vi "Alligent.vi"() -> ()   [LabVIEW 2018]
uses:
  <vilib>/userdefined/High Color/IMAQdx.ctl
  <vilib>/Utility/miscctls.llb/LVRowAndColumnTypeDef.ctl
  <vilib>/vision/driver/NI_Vision_Acquisition_Software.lvlib
  <vilib>/vision/NI_Vision_Development_Module.lvlib
panel:
  out "Centroid":cluster{"X Centroid":sgl, "Y Centroid":sgl} {"Y Centroid" format="%.2f"; "X Centroid" format="%.2f"}
  in  "观察位置":bool
  in  "记录位置":bool
  out "运行提示":string
  in  "相机曝光时间/ms":dbl(slide) scale=0.0..1000.0
  in  "俯仰":cluster{"前进0.1":bool, "后退0.1":bool, "目标位置":dbl} {"目标位置" max=0.0}
  in  "Z":cluster{"前进1mm":bool, "后退1mm":bool, "目标位置":dbl} {"目标位置" max=0.0}
  in  "Y":cluster{"前进1mm":bool, "后退1mm":bool, "目标位置":dbl} {"目标位置" max=0.0}
  in  "X":cluster{"前进1mm":bool, "后退1mm":bool, "目标位置":dbl} {"目标位置" max=0.0}
  in  "退出":bool
  in  "衰减挡位":T1 scale=0.0..3.0
  out "激光器状态":i32[](listbox)
  in  "初始位置":bool
  in  "链接电机":bool
  in  "链接相机":bool
  out "近场图":T2(plugin-control)
  in  "旋转":T3 {"目标位置" max=0.0}
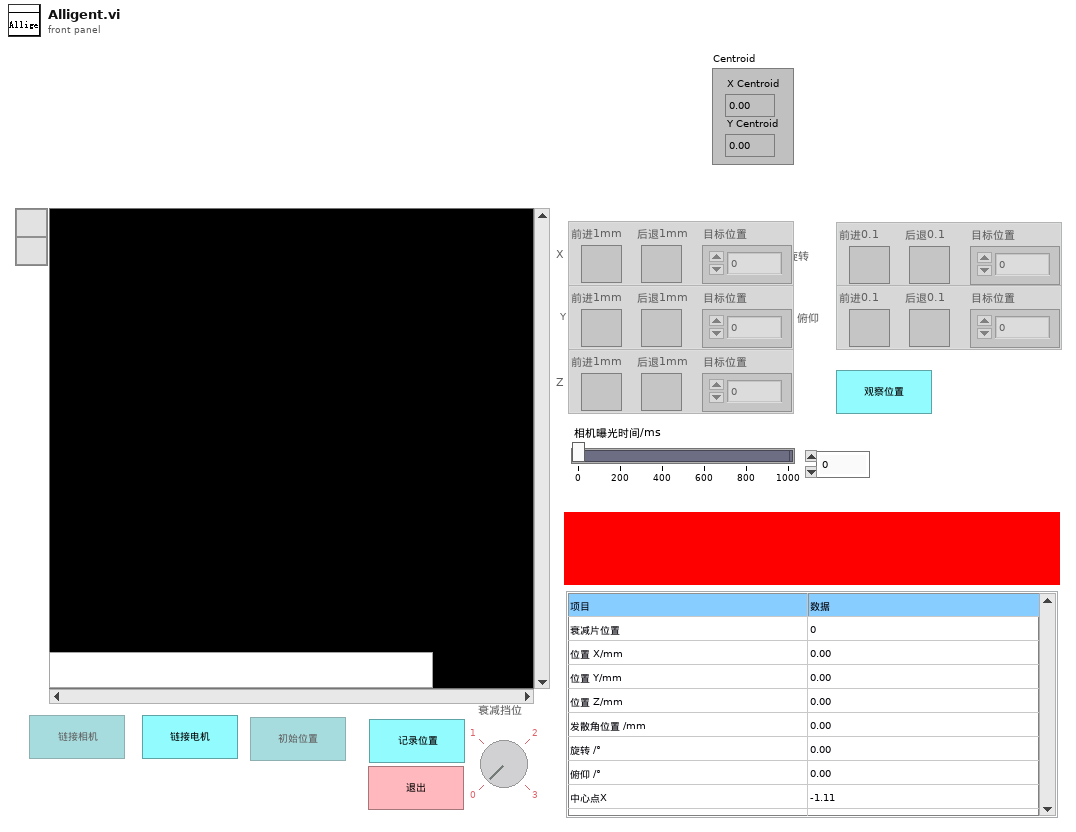
[diagram p1: front panel]
types:
  T1 = typedef "衰减片前面板.ctl" = u8
  T2 = typedef "IMAQ Image.ctl" = refnum<image>
  T3 = typedef "位置调整控件.ctl" = cluster{"前进0.1":bool, "后退0.1":bool, "目标位置":dbl}
  T4 = typedef "IMAQdx.ctl" = refnum<k21>
  T5 = cluster{"链接相机":refnum<vi>, "链接电机":refnum<vi>, "初始位置":refnum<vi>, "退出":refnum<vi>, "衰减挡位":refnum<vi>, "相机曝光时间/ms":refnum<vi>}
  T6 = cluster{"X":refnum<vi>, " Y":refnum<vi>, "Z":refnum<vi>, "  旋转":refnum<vi>, "俯仰":refnum<vi>, "观察位置":refnum<vi>}
  T7 = typedef "衰减片电机位置枚举器.ctl" = enum16{"0倍", "10倍", "100倍", "1000倍"}
  T8 = enum8{"Enabled", "Disabled", "Disabled and Grayed Out"}
  T9 = typedef "衰减片电机指令枚举器.ctl" = enum16{"归0", "停止", "运动", "轴设置", "通信连接", "读取位置"}
  T10 = typedef "控制电机指令枚举器.ctl" = enum16{"归0", "停止", "运动", "轴设置", "通信连接"}
  T11 = typedef "衰减片电机枚举.ctl" = enum16{"小积分球衰减", "偏振仪衰减", "近场相机衰减", "远场相机衰减"}
  T12 = typedef "控制电机位置枚举器.ctl" = enum16{"远场扫描", "发散角扫描", "远场相机", "近场相机", "时间波形", "偏振", "能量", "功率", "光谱"}
  T13 = typedef "控制电机枚举器.ctl" = enum16{"Z", "Y", "X", "发散角", "俯仰", "旋转"}
  T14 = cluster{"激光器型号":string, "X":dbl, "Y":dbl, "Z":dbl, "Rotate":dbl, "Pitching":dbl, "DivergeAngle":dbl, "衰减片位置":cluster{"小积分球位置":T7, "偏振仪位置 ":T7, "近场相机位置 ":T7, "远场相机位置":T7}, "Type":string, "Serial":string}
  T15 = cluster{"远场相机":cluster{"控制电机":T13, "位置":dbl}[], "近场相机":cluster{"控制电机":T13, "位置":dbl}[], "时间波形":cluster{"控制电机":T13, "位置":dbl}[], "偏振":cluster{"控制电机":T13, "位置":dbl}[], "能量":cluster{"控制电机":T13, "位置":dbl}[], "功率":cluster{"控制电机":T13, "位置":dbl}[], "光谱":cluster{"控制电机":T13, "位置":dbl}[], "准直光焦点":cluster{"控制电机":T13, "位置":dbl}[]}
  T16 = typedef "LVRowAndColumnTypeDef.ctl" = cluster{"Row":i32, "Column":i32}
  T17 = cluster{cluster{"控制电机":T13, "NewVal":dbl}, "CMD":string}
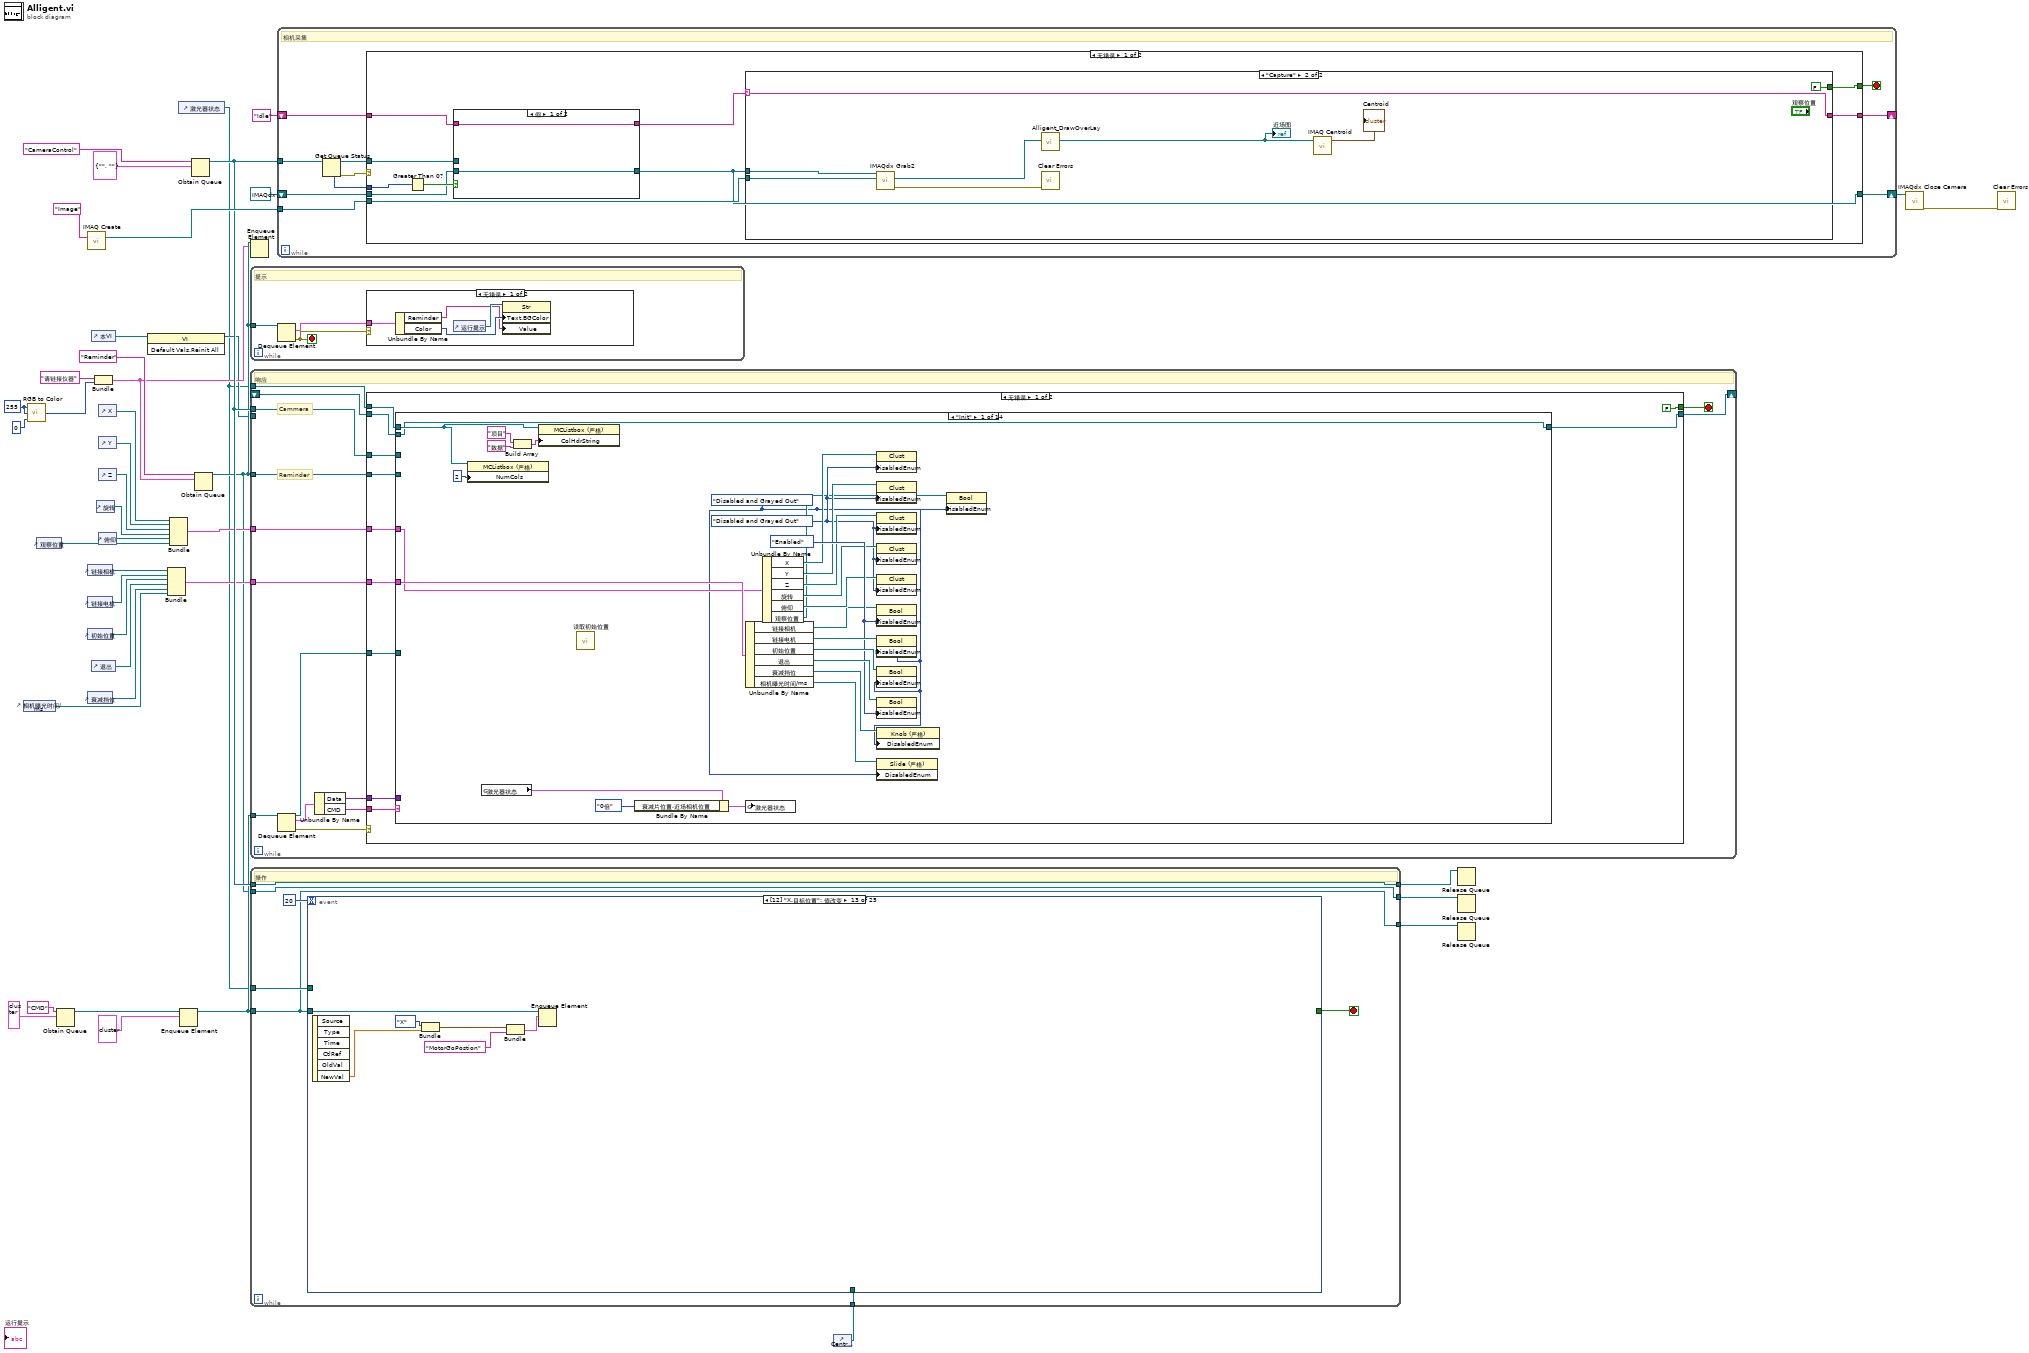
[diagram p0: block diagram]
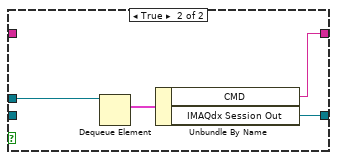
[diagram p3: hidden frame]
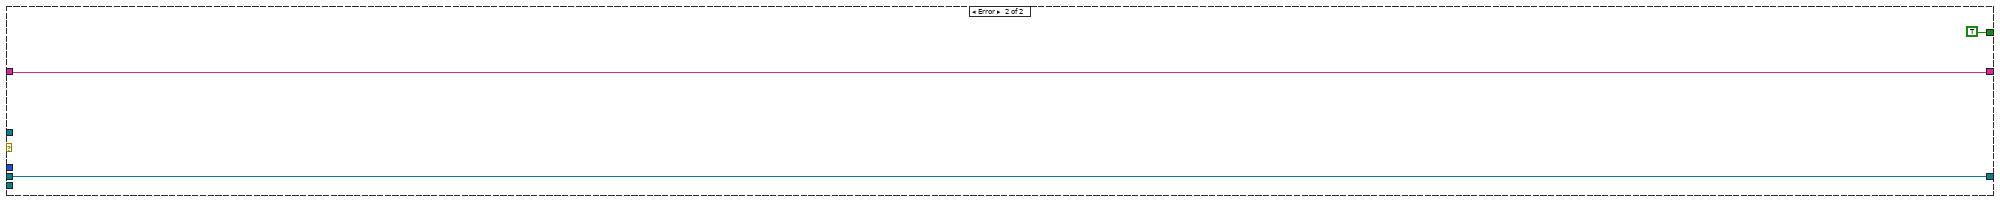
[diagram p5: hidden frame]
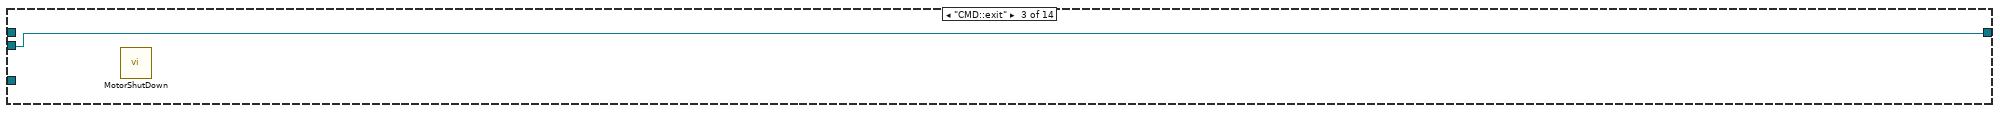
[diagram p7: hidden frame]
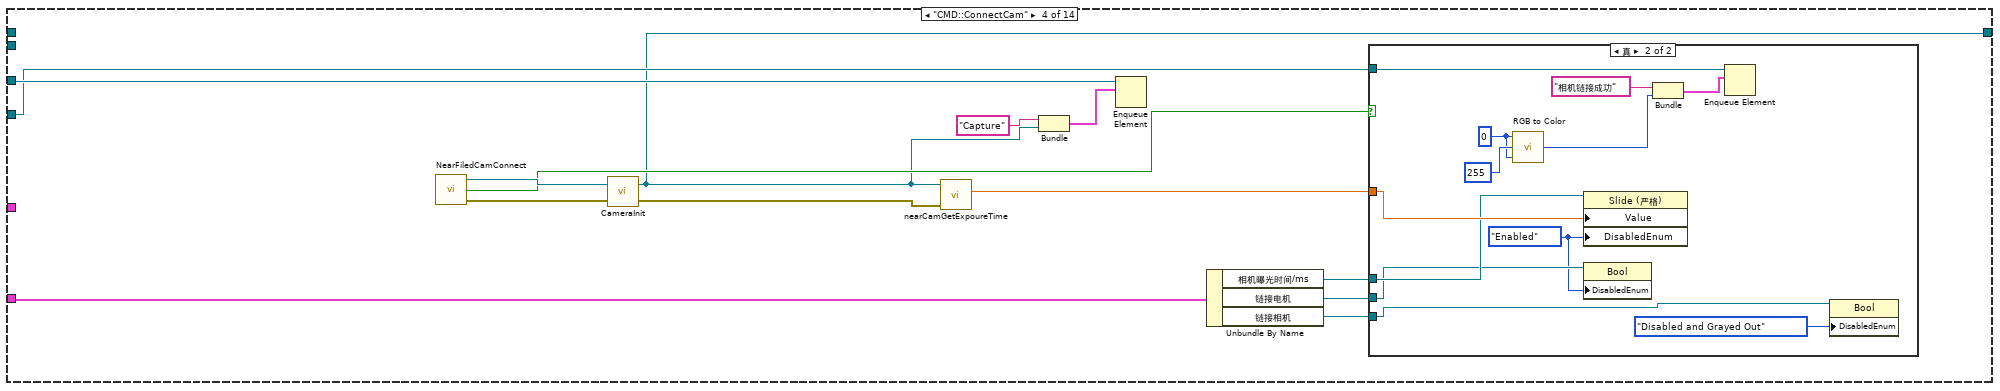
[diagram p8: hidden frame]
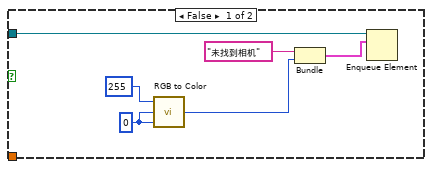
[diagram p9: hidden frame]
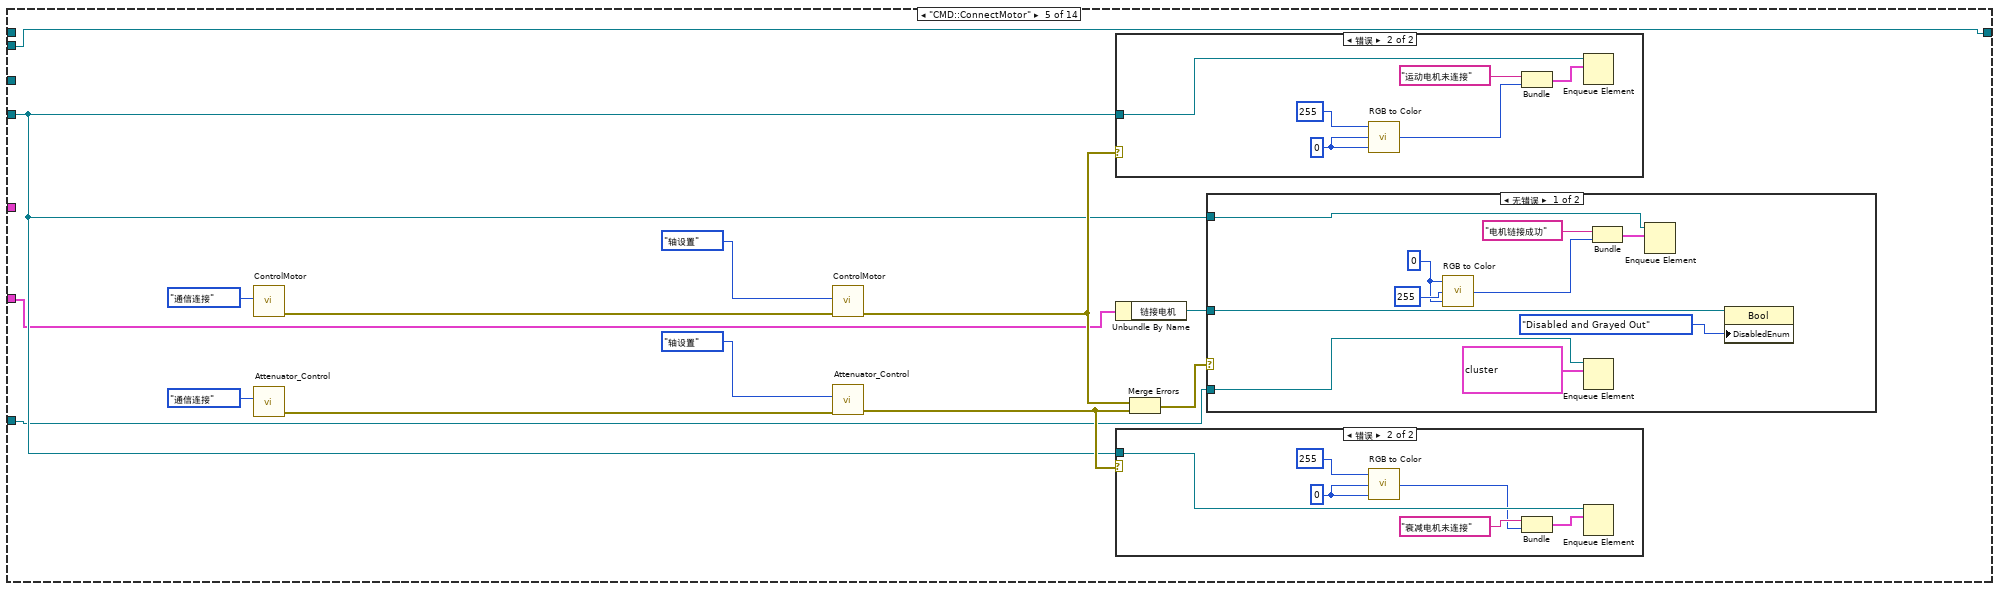
[diagram p10: hidden frame]
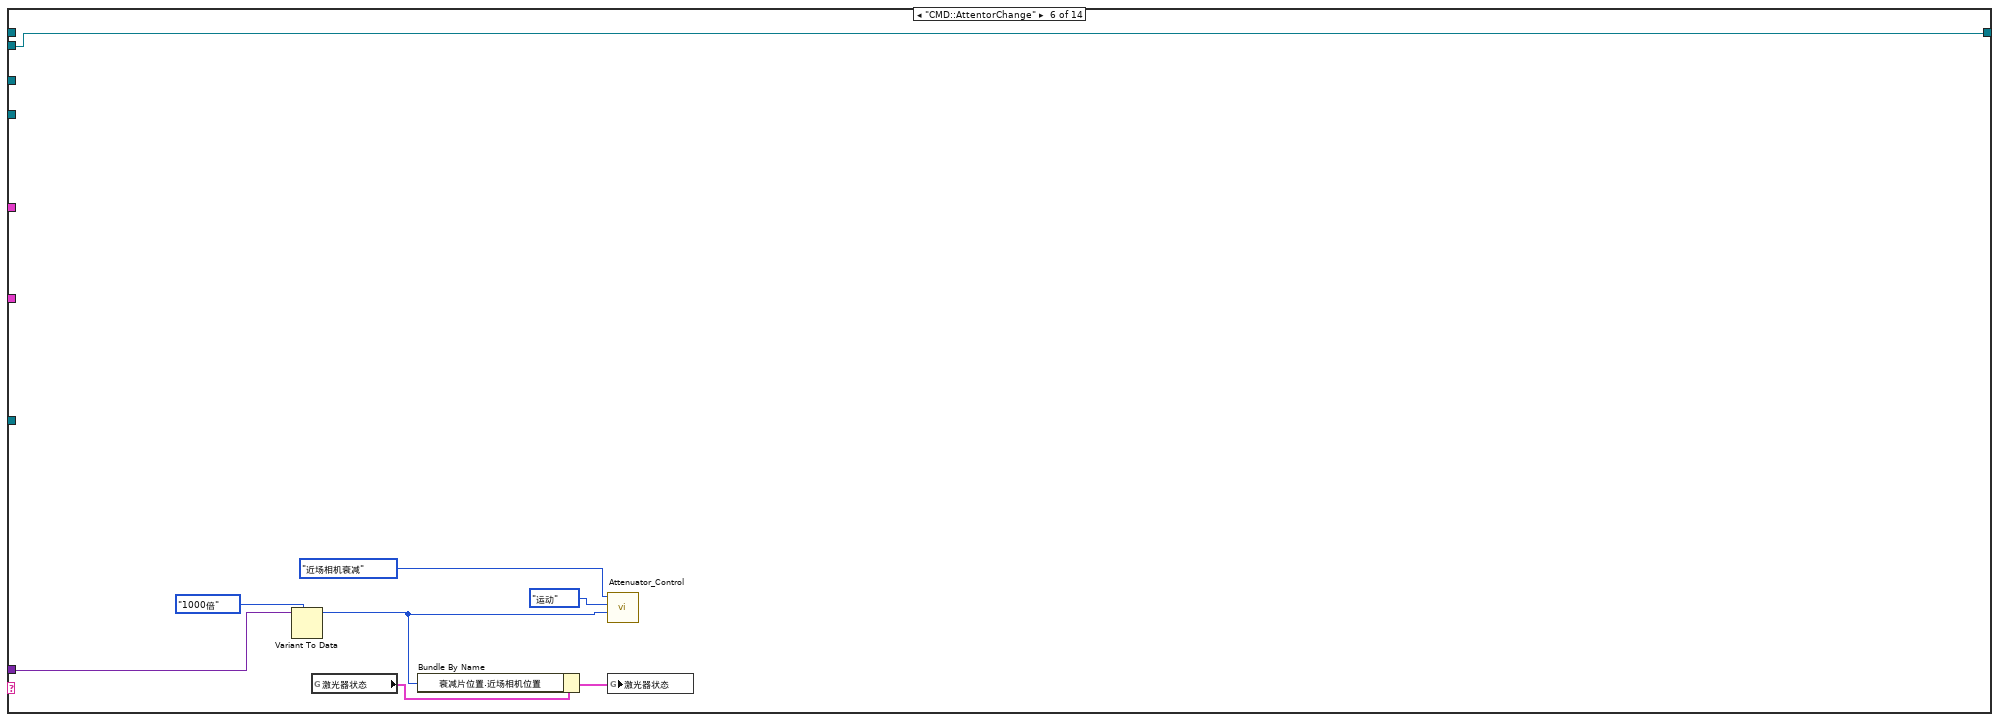
[diagram p14: hidden frame]
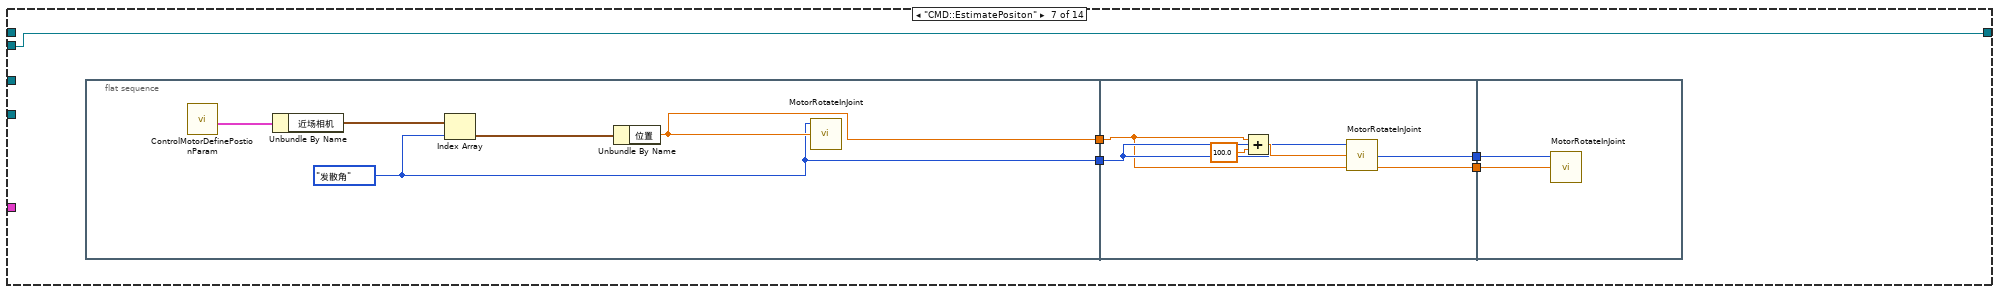
[diagram p15: hidden frame]
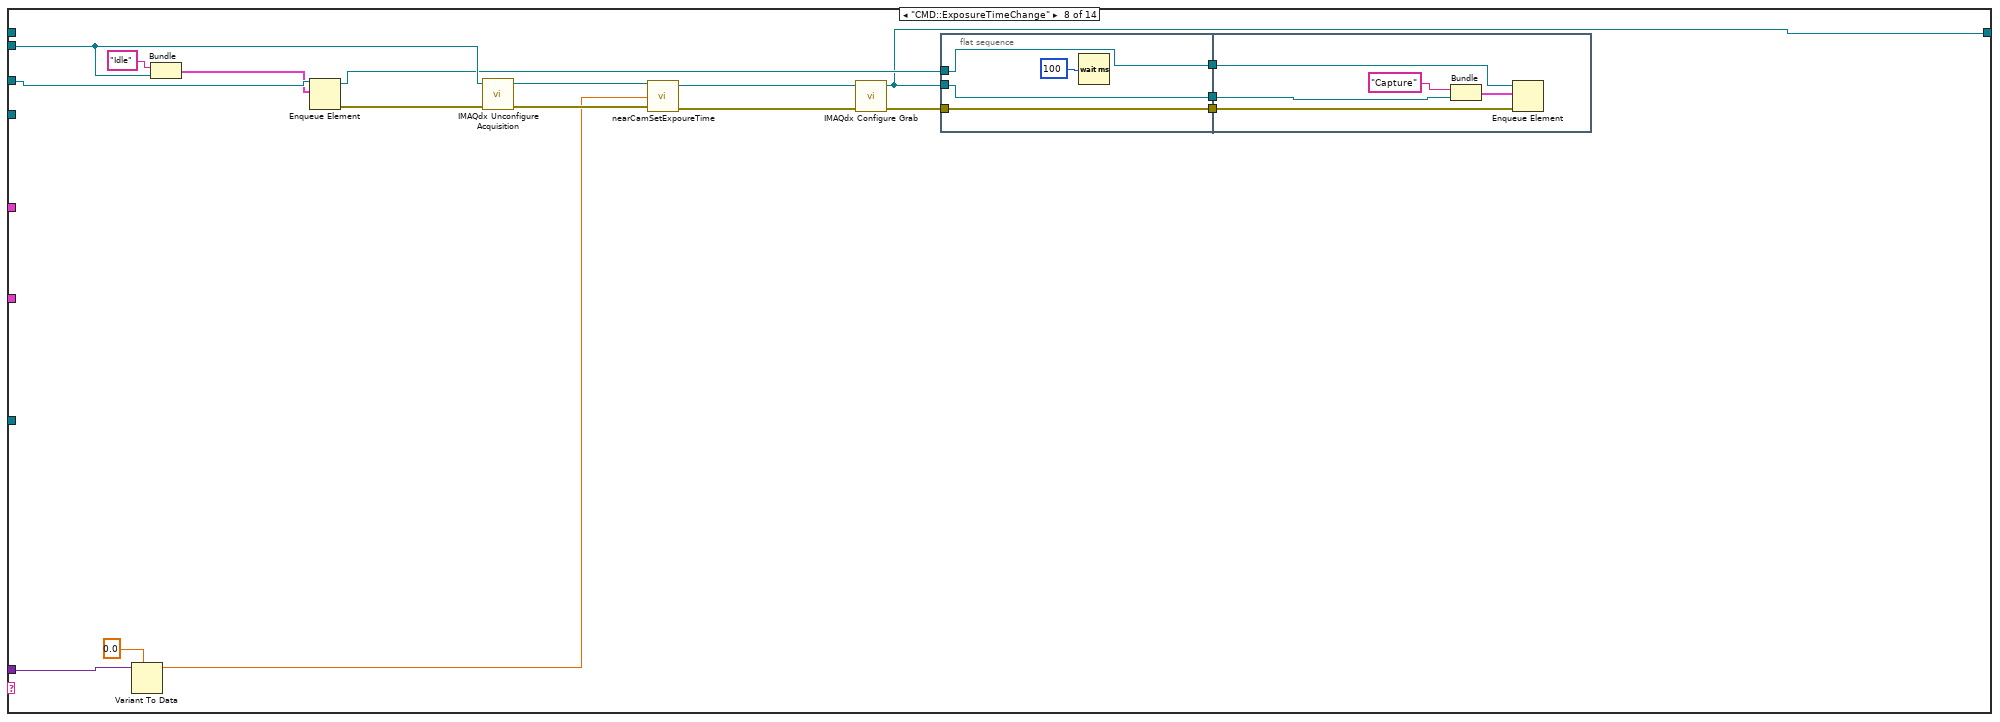
[diagram p16: hidden frame]
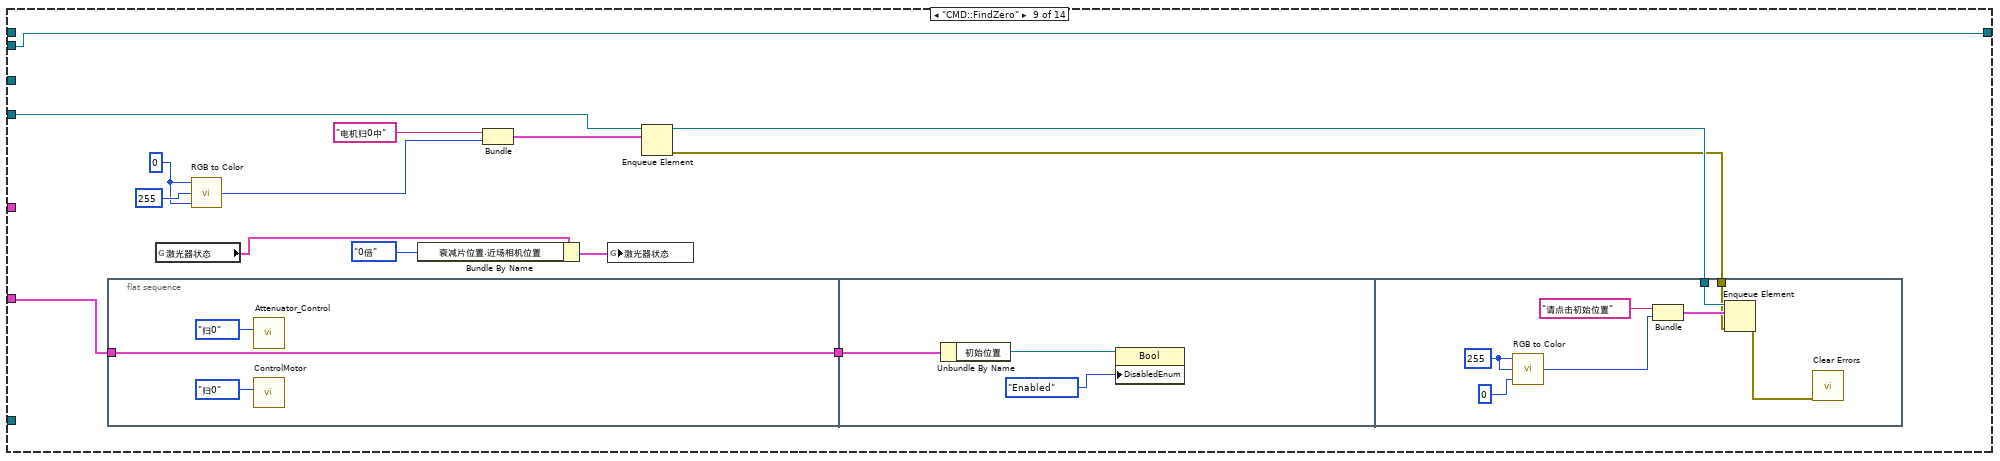
[diagram p17: hidden frame]
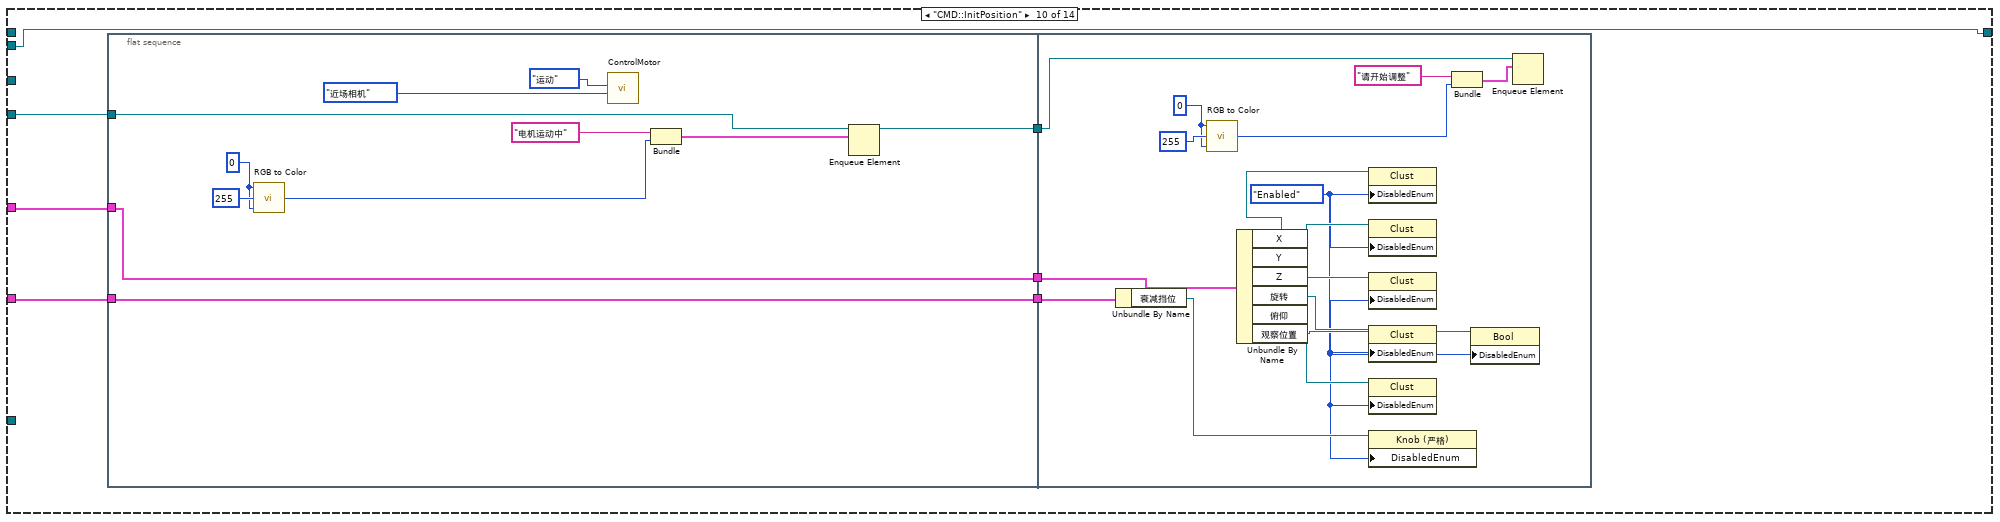
[diagram p18: hidden frame]
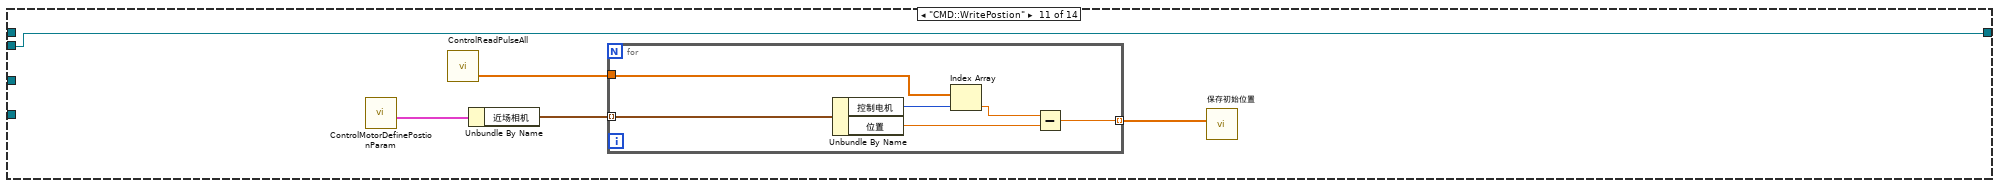
[diagram p19: hidden frame]
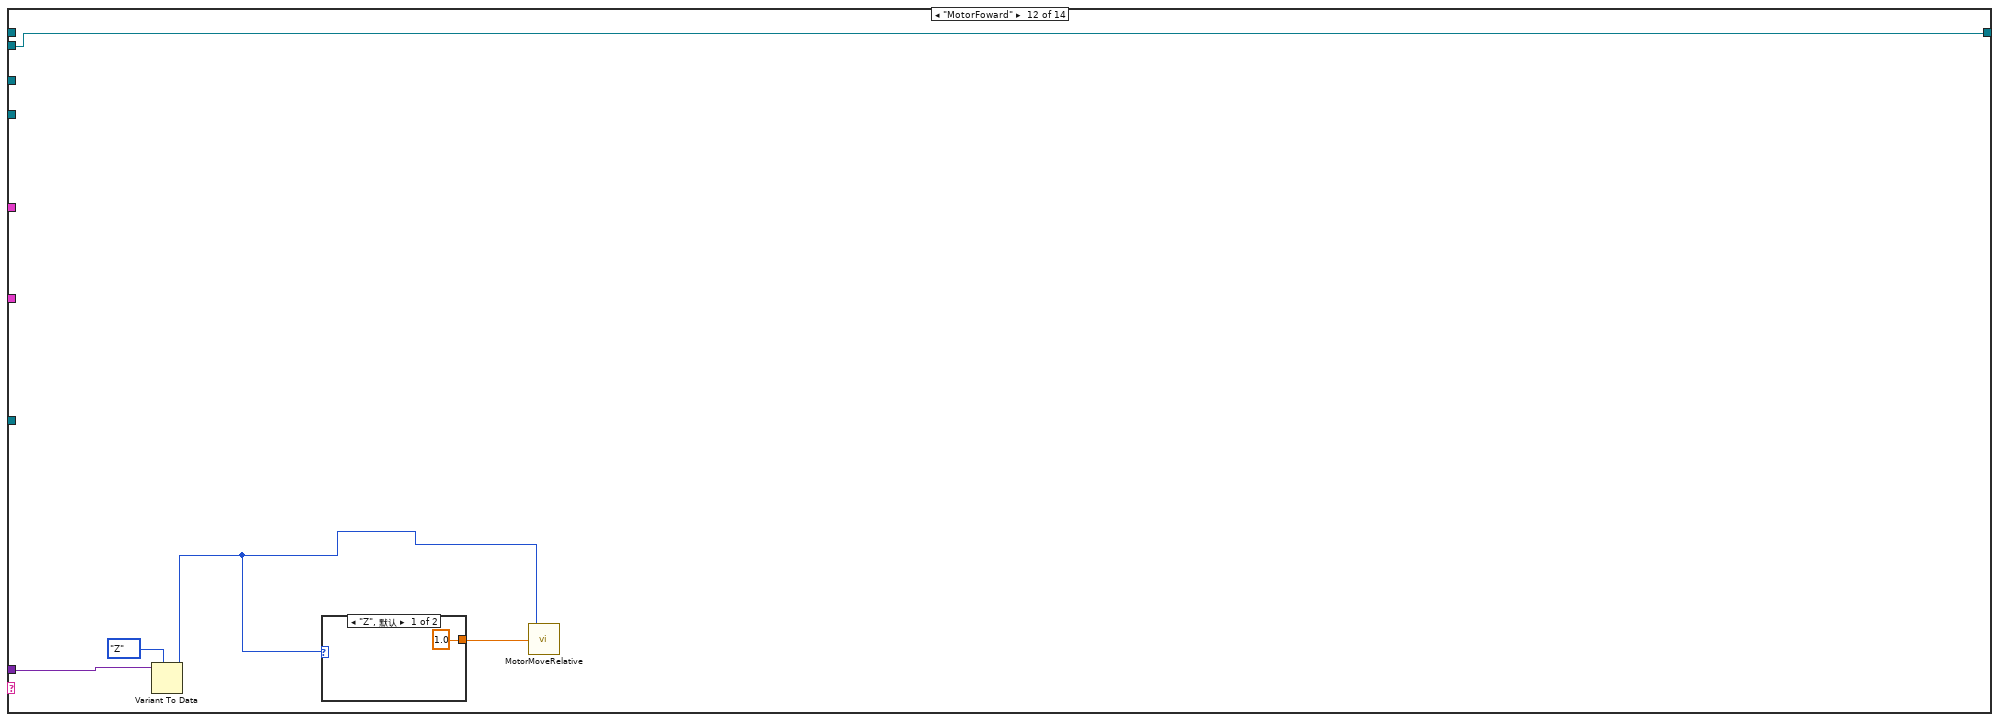
[diagram p20: hidden frame]
diagram:
  w8 = 255
  n1 = control-ref of="相机曝光时间/ms"() -> (w6:refnum<vi>)
  n2 = call <vilib>:"RGB to Color.vi"("B"=0, "G"=w8, "R"=w8) -> ("Color"=w31:u32)
  n3 = control-ref of="观察位置"() -> (w1:refnum<vi>)
  n4 = Obtain Queue(name (unnamed)="CMD" ("名称（未命名）"), element data type=cluster{"Data":variant, "CMD":string} {"Data"=variant, "CMD"=""}) -> (queue out=w39:refnum<queue>)  [unwired: 3 in, 2 out]
  n5 = call "IMAQ Create"("Image Name"="Image") -> ("New Image"=w33:T2)  [unwired: 4 in, 1 out]
  n6 = control-ref of="链接相机"() -> (w27:refnum<vi>)
  n7 = control-ref of="链接电机"() -> (w26:refnum<vi>)
  n8 = control-ref of="初始位置"() -> (w25:refnum<vi>)
  n9 = control-ref of="衰减挡位"() -> (w23:refnum<vi>)
  n10 = control-ref of="本VI"() -> (w5:refnum<vi>)
  n11 = control-ref of="退出"() -> (w24:refnum<vi>)
  n12 = Bundle("Reminder"="请链接仪器", "Color"=w31) -> (w11:cluster{"Reminder":string, "Color":u32})  [unwired: 1 in]
  n13 = control-ref of="旋转"() -> (w20:refnum<vi>)
  n14 = control-ref of="X"() -> (w22:refnum<vi>)
  n15 = control-ref of="Y"() -> (w18:refnum<vi>)
  n16 = control-ref of="Z"() -> (w21:refnum<vi>)
  n17 = control-ref of="俯仰"() -> (w19:refnum<vi>)
  n18 = invoke class="VI" method="Default Vals.Reinit All"(reference=w5) -> (reference out=w4:refnum<vi>)  [unwired: 2 in, 2 out]
  n19 = Bundle("链接相机"=w27, "链接电机"=w26, "初始位置"=w25, "退出"=w24, "衰减挡位"=w23, "相机曝光时间/ms"=w6) -> (w15:T5)  [unwired: 1 in]
  n20 = Bundle("X"=w22, "Y"=w18, "Z"=w21, "旋转"=w20, "俯仰"=w19, "观察位置"=w1) -> (w14:T6)  [unwired: 1 in]
  n21 = control-ref of="激光器状态"() -> (w3:refnum<vi>)
  n22 = Enqueue Element(queue=w39, element=cluster{"Data":variant, "CMD":string} {"Data"=variant, "CMD"="Init"}) -> (queue out=w17:refnum<queue>)  [unwired: 2 in, 2 out]
  n23 = Obtain Queue(name (unnamed)="CameraControl" ("名称（未命名）"), element data type=cluster{"CMD":string, "IMAQdx Session Out":T4} {"CMD"="", "IMAQdx Session Out"=""}) -> (queue out=w30:refnum<queue>)  [unwired: 3 in, 2 out]
  n24 = Obtain Queue(name (unnamed)="Reminder" ("Reminder"), element data type=w11) -> (queue out=w13:refnum<queue>)  [unwired: 3 in, 2 out]
  n25 = Enqueue Element(queue=w13, element=w11) -> ()  [unwired: 2 in, 3 out]
  n26 = while "While循环" {
    tunnel: w13 -> [w45]
    stop <- w44 stop-if-true
    # "提示"
    n27 = Dequeue Element(queue=w45) -> (element=w43:cluster{"Reminder":string, "Color":u32}, error out=w44:errorcluster)  [unwired: 2 in, 2 out]
    n28 = case shown="无错误" w44 {
      tunnel: w43 -> [w48 _]
      frame No Error {
        n29 = Unbundle By Name(w48) -> ("Reminder"=w46:string, "Color"=w47:u32)
        n30 = control-ref of="运行提示"() -> (w49:refnum<vi>)
        n31 = property class="Str"(reference=w49, "Text.BGColor"=w47, "Value"=w46) -> ()  [unwired: 1 in, 2 out]
      }
      frame Error {
      }
    }
  }
  n32 = while "While循环" {
    tunnel: w17 -> [w59]
    tunnel: w30 -> [w58]
    tunnel: w13 -> [w57]
    tunnel: w15 -> [w56]
    tunnel: w14 -> [w55]
    shift-right: [w53] -> _
    shift-left: _ -> [w52]
    tunnel: w3 -> [w51]
    tunnel: w4 -> [_]
    stop <- w62 stop-if-true
    # "Cammera"
    # "Reminder"
    # "响应"
    n33 = Dequeue Element(queue=w59) -> (queue out=w50:refnum<queue>, element=w61:cluster{"Data":variant, "CMD":string}, error out=w63:errorcluster)  [unwired: 2 in, 1 out]
    n34 = Unbundle By Name(w61) -> ("Data"=w54:variant, "CMD"=w60:string)
    n35 = case shown="无错误" w63 {
      tunnel: [FALSE TRUE] -> w62
      tunnel: w60 -> [w73 _]
      tunnel: w58 -> [w72 _]
      tunnel: w57 -> [w71 _]
      tunnel: w56 -> [w70 _]
      tunnel: w55 -> [w69 _]
      tunnel: w54 -> [w68 _]
      tunnel: [w67 w315] -> w53
      tunnel: w52 -> [w66 w315]
      tunnel: w51 -> [w65 _]
      tunnel: w50 -> [w64 _]
      frame No Error {
        n36 = case shown="\"Init\"" w73 {
          tunnel: w72 -> [_ _ _ w114 _ _ _ w210 _ _ _ _ _ _]
          tunnel: w71 -> [_ _ _ w110 w139 _ _ _ w227 w252 _ _ _ _]
          tunnel: w70 -> [w95 _ _ w106 w136 _ _ _ w235 w256 _ _ _ _]
          tunnel: w69 -> [w89 _ _ _ _ _ _ _ _ w253 _ _ _ _]
          tunnel: w68 -> [_ _ _ _ _ w176 _ w211 _ _ _ w299 w303 w311]
          tunnel: [w78 w101 w102 w109 w137 w171 w181 w208 w223 w250 w288 w296 w302 w307] -> w67
          tunnel: w66 -> [w78 w101 w102 _ w137 w171 w181 w212 w223 w250 w288 w296 w302 w307]
          tunnel: w65 -> [w79 _ _ _ _ _ _ _ _ _ _ _ _ _]
          tunnel: w64 -> [_ _ _ _ w138 _ _ _ _ _ _ _ _ _]
          frame "Init" {
            w88 = T8."Disabled and Grayed Out" ("禁用")
            w96 = T8."Enabled" ("禁用")
            w75 = T8."Disabled and Grayed Out" ("禁用")
            n37 = property on="属性节点" class="MCListbox (严格)"(reference=w79, "NumCols"=u32 2 ("列数")) -> ()  [unwired: 1 in, 2 out]
            n38 = global read "参数.vi" "激光器状态"() -> (w86:T14)
            n39 = Build Array("项目", "数据") -> (w80:string[])
            n40 = property on="属性节点" class="MCListbox (严格)"(reference=w79, "ColHdrString"=w80) -> ()  [unwired: 1 in, 2 out]
            n41 = call "读取初始位置.vi"() -> ()  [unwired: 11 in, 1 out]
            n42 = Bundle By Name(cluster=w86, "衰减片位置.近场相机位置"=衰减片电机位置枚举器."0倍") -> (w84:T14)
            n43 = Unbundle By Name(w95) -> ("链接相机"=w87:refnum<vi>, "链接电机"=w97:refnum<vi>, "初始位置"=w98:refnum<vi>, "退出"=w99:refnum<vi>, "衰减挡位"=w100:refnum<vi>, "相机曝光时间/ms"=w77:refnum<vi>)
            n44 = global write "参数.vi" "激光器状态"(w84) -> ()
            n45 = Unbundle By Name(w89) -> ("X"=w90:refnum<vi>, "Y"=w91:refnum<vi>, "Z"=w92:refnum<vi>, "旋转"=w93:refnum<vi>, "俯仰"=w94:refnum<vi>, "观察位置"=w76:refnum<vi>)
            n46 = property class="Clust"(reference=w90, "DisabledEnum"=w88) -> ()  [unwired: 1 in, 2 out]
            n47 = property class="Clust"(reference=w91, "DisabledEnum"=w88) -> ()  [unwired: 1 in, 2 out]
            n48 = property class="Clust"(reference=w92, "DisabledEnum"=w88) -> ()  [unwired: 1 in, 2 out]
            n49 = property class="Clust"(reference=w93, "DisabledEnum"=w88) -> ()  [unwired: 1 in, 2 out]
            n50 = property class="Clust"(reference=w94, "DisabledEnum"=w88) -> ()  [unwired: 1 in, 2 out]
            n51 = property class="Bool"(reference=w87, "DisabledEnum"=w96) -> ()  [unwired: 1 in, 2 out]
            n52 = property class="Bool"(reference=w97, "DisabledEnum"=w75) -> ()  [unwired: 1 in, 2 out]
            n53 = property class="Bool"(reference=w98, "DisabledEnum"=w75) -> ()  [unwired: 1 in, 2 out]
            n54 = property class="Bool"(reference=w99, "DisabledEnum"=w96) -> ()  [unwired: 1 in, 2 out]
            n55 = property class="Knob (严格)"(reference=w100, "DisabledEnum"=w75) -> ()  [unwired: 1 in, 2 out]
            n56 = property class="Slide (严格)"(reference=w77, "DisabledEnum"=w75) -> ()  [unwired: 1 in, 2 out]
            n57 = property class="Bool"(reference=w76, "DisabledEnum"=w75) -> ()  [unwired: 1 in, 2 out]
          }
          frame "Idle", Default {
          }
          frame "CMD::exit" {
            n58 = call "MotorShutDown.vi"() -> ()  [unwired: 11 in, 1 out]
          }
          frame "CMD::ConnectCam" {
            n59 = call "NearFiledCamConnect.vi"() -> ("Session Out"=w116:T4, "连接状态"=w111:bool, "错误输出"=w115:errorcluster)  [unwired: 2 in]
            n60 = call "CameraInit.vi"("错误输入（无错误）"=w115, "IMAQdx Session"=w116) -> ("error out"=w107:errorcluster, "IMAQdx Session Out"=w109:T4)
            n61 = call "nearCamGetExpoureTime.vi"("错误输入（无错误）"=w107, "IMAQdx Session"=w109) -> ("TimeOut"=w108:dbl)  [unwired: 2 in, 4 out]
            n62 = Bundle("Capture", "IMAQdx Session Out"=w109) -> (w112:cluster{string, "IMAQdx Session Out":T4})  [unwired: 1 in]
            n63 = Enqueue Element(queue=w114, element=w112) -> ()  [unwired: 2 in, 3 out]
            n64 = Unbundle By Name(w106) -> ("相机曝光时间/ms"=w105:refnum<vi>, "链接电机"=w104:refnum<vi>, "链接相机"=w103:refnum<vi>)
            n65 = case shown="真" w111 {
              tunnel: w110 -> [w122 w129]
              tunnel: w108 -> [_ w128]
              tunnel: w105 -> [_ w127]
              tunnel: w104 -> [_ w126]
              tunnel: w103 -> [_ w124]
              frame False {
                w121 = 0
                n66 = call <vilib>:"RGB to Color.vi"("B"=w121, "G"=w121, "R"=u8 255) -> ("Color"=w118:u32)
                n67 = Bundle("未找到相机", "Color"=w118) -> (w117:cluster{string, "Color":u32})  [unwired: 1 in]
                n68 = Enqueue Element(queue=w122, element=w117) -> ()  [unwired: 2 in, 3 out]
              }
              frame True {
                w125 = T8."Enabled" ("禁用")
                w130 = 0
                n69 = call <vilib>:"RGB to Color.vi"("B"=w130, "G"=u8 255 ("R"), "R"=w130) -> ("Color"=w133:u32)
                n70 = property class="Slide (严格)"(reference=w127, "Value"=w128, "DisabledEnum"=w125) -> ()  [unwired: 1 in, 2 out]
                n71 = property class="Bool"(reference=w126, "DisabledEnum"=w125) -> ()  [unwired: 1 in, 2 out]
                n72 = Bundle("相机链接成功", "Color"=w133) -> (w132:cluster{string, "Color":u32})  [unwired: 1 in]
                n73 = Enqueue Element(queue=w129, element=w132) -> ()  [unwired: 2 in, 3 out]
                n74 = property class="Bool"(reference=w124, "DisabledEnum"=T8."Disabled and Grayed Out" ("禁用")) -> ()  [unwired: 1 in, 2 out]
              }
            }
          }
          frame "CMD::ConnectMotor" {
            n75 = call "ControlMotor.vi"("控制电机指令"=控制电机指令枚举器."通信连接") -> ("错误输出 2"=w147:errorcluster)  [unwired: 7 in]
            n76 = call "Attenuator_Control.vi"("控制电机指令"=衰减片电机指令枚举器."通信连接") -> ("error out"=w145:errorcluster)  [unwired: 4 in, 1 out]
            n77 = call "ControlMotor.vi"("控制电机指令"=控制电机指令枚举器."轴设置", "错误输入"=w147) -> ("错误输出 2"=w142:errorcluster)  [unwired: 6 in]
            n78 = call "Attenuator_Control.vi"("错误输入"=w145, "控制电机指令"=衰减片电机指令枚举器."轴设置") -> ("error out"=w141:errorcluster)  [unwired: 3 in, 1 out]
            n79 = case shown="错误" w142 {
              tunnel: w139 -> [_ w170]
              frame No Error {
              }
              frame Error {
                w169 = 0
                n80 = call <vilib>:"RGB to Color.vi"("B"=w169, "G"=w169, "R"=u8 255) -> ("Color"=w166:u32)
                n81 = Bundle("运动电机未连接", "Color"=w166) -> (w165:cluster{string, "Color":u32})  [unwired: 1 in]
                n82 = Enqueue Element(queue=w170, element=w165) -> ()  [unwired: 2 in, 3 out]
              }
            }
            n83 = Unbundle By Name(w136) -> ("链接电机"=w135:refnum<vi>)
            n84 = case shown="错误" w141 {
              tunnel: w139 -> [_ w164]
              frame No Error {
              }
              frame Error {
                w163 = 0
                n85 = call <vilib>:"RGB to Color.vi"("B"=w163, "G"=w163, "R"=u8 255) -> ("Color"=w160:u32)
                n86 = Bundle("衰减电机未连接", "Color"=w160) -> (w159:cluster{string, "Color":u32})  [unwired: 1 in]
                n87 = Enqueue Element(queue=w164, element=w159) -> ()  [unwired: 2 in, 3 out]
              }
            }
            n88 = Merge Errors(w142, w141) -> (w140:errorcluster)
            n89 = case shown="无错误" w140 {
              tunnel: w139 -> [w153 _]
              tunnel: w138 -> [w151 _]
              tunnel: w135 -> [w149 _]
              frame No Error {
                w154 = 0
                n90 = call <vilib>:"RGB to Color.vi"("B"=w154, "G"=u8 255 ("R"), "R"=w154) -> ("Color"=w157:u32)
                n91 = Enqueue Element(queue=w151, element=cluster{"Data":variant, "CMD":string} {"Data"=variant, "CMD"="CMD::FindZero"} ("元素")) -> ()  [unwired: 2 in, 3 out]
                n92 = Bundle("电机链接成功", "Color"=w157) -> (w156:cluster{string, "Color":u32})  [unwired: 1 in]
                n93 = Enqueue Element(queue=w153, element=w156) -> ()  [unwired: 2 in, 3 out]
                n94 = property class="Bool"(reference=w149, "DisabledEnum"=T8."Disabled and Grayed Out" ("禁用")) -> ()  [unwired: 1 in, 2 out]
              }
              frame Error {
              }
            }
          }
          frame "CMD::AttentorChange" {
            n95 = Variant To Data(type=衰减片电机位置枚举器."1000倍" ("位置"), Variant=w176) -> (data=w173:T7)  [unwired: 1 in, 1 out]
            n96 = global read "参数.vi" "激光器状态"() -> (w174:T14)
            n97 = Bundle By Name(cluster=w174, "衰减片位置.近场相机位置"=w173) -> (w172:T14)
            n98 = call "Attenuator_Control.vi"("位置"=w173, "控制电机指令"=衰减片电机指令枚举器."运动", "电机"=衰减片电机枚举."近场相机衰减") -> ()  [unwired: 2 in, 2 out]
            n99 = global write "参数.vi" "激光器状态"(w172) -> ()
          }
          frame "CMD::EstimatePositon" {
            n100 = flat-sequence {
              tunnel: [w185] -> w183
              tunnel: [w184] -> w182
              tunnel: w183 -> [w189]
              tunnel: w182 -> [w190]
              tunnel: [w190] -> w180
              tunnel: [w189] -> w179
              tunnel: w180 -> [w194]
              tunnel: w179 -> [w193]
              frame #0 {
                w184 = 控制电机枚举器."发散角" ("控制电机")
                n101 = call "ControlMotorDefinePostionParam.vi"() -> ("位置信息"=w188:T15)  [unwired: 11 in]
                n102 = Unbundle By Name(w188) -> ("近场相机"=w187:cluster{"控制电机":T13, "位置":dbl}[])
                n103 = Index Array(array=w187, index=w184) -> (element=w186:cluster{"控制电机":T13, "位置":dbl})
                n104 = Unbundle By Name(w186) -> ("位置"=w185:dbl)
                n105 = call "MotorRotateInJoint.vi"("位置"=w185, "axis"=w184) -> ()  [unwired: 2 in, 1 out]
              }
              frame #1 {
                n106 = Add(x=w189, y=100.0) -> (x+y=w191:dbl)
                n107 = call "MotorRotateInJoint.vi"("位置"=w191, "axis"=w190) -> ()  [unwired: 2 in, 1 out]
              }
              frame #2 {
                n108 = call "MotorRotateInJoint.vi"("位置"=w193, "axis"=w194) -> ()  [unwired: 2 in, 1 out]
              }
            }
          }
          frame "CMD::ExposureTimeChange" {
            n109 = Variant To Data(type=0.0 ("Time/us"), Variant=w211) -> (data=w200:dbl)  [unwired: 1 in, 1 out]
            n110 = Bundle("CMD"="Idle", "Session Out"=w212) -> (w206:cluster{"CMD":string, "Session Out":T4})  [unwired: 1 in]
            n111 = Enqueue Element(queue=w210, element=w206) -> (queue out=w209:refnum<queue>, error out=w199:errorcluster)  [unwired: 2 in, 1 out]
            n112 = call <vilib>:"IMAQdx Unconfigure Acquisition.vi"("error in"=w199, "Session In"=w212) -> ("error out"=w204:errorcluster, "Session Out"=w205:T4)  [unwired: 8 in]
            n113 = call "nearCamSetExpoureTime.vi"("错误输入（无错误）"=w204, "Time/us"=w200, "IMAQdx Session"=w205) -> ("错误输出"=w202:errorcluster, "IMAQdx Session Out"=w203:T4)  [unwired: 1 in, 3 out]
            n114 = call <vilib>:"IMAQdx Configure Grab.vi"("error in"=w202, "Session In"=w203) -> ("error out"=w198:errorcluster, "Session Out"=w208:T4)  [unwired: 8 in]
            n115 = flat-sequence {
              tunnel: w198 -> [w214]
              tunnel: w208 -> [w215]
              tunnel: w209 -> [w216]
              tunnel: [w216] -> w197
              tunnel: [w215] -> w196
              tunnel: [w214] -> w195
              tunnel: w197 -> [w221]
              tunnel: w196 -> [w220]
              tunnel: w195 -> [w217]
              frame #0 {
                n116 = Wait (ms)(milliseconds to wait=u32 100 ("等待时间（毫秒）")) -> ()  [unwired: 1 out]
              }
              frame #1 {
                n117 = Bundle("CMD"="Capture", "Session Out"=w220) -> (w218:cluster{"CMD":string, "Session Out":T4})  [unwired: 1 in]
                n118 = Enqueue Element(queue=w221, element=w218, error in (no error)=w217) -> ()  [unwired: 1 in, 3 out]
              }
            }
          }
          frame "CMD::FindZero" {
            w225 = 0
            n119 = flat-sequence {
              tunnel: w235 -> [w236]
              tunnel: [w236] -> w234
              tunnel: w234 -> [w241]
              tunnel: w224 -> [w246]
              tunnel: w222 -> [w243]
              frame #0 {
                n120 = call "Attenuator_Control.vi"("控制电机指令"=衰减片电机指令枚举器."归0") -> ()  [unwired: 4 in, 2 out]
                n121 = call "ControlMotor.vi"("控制电机指令"=控制电机指令枚举器."归0") -> ()  [unwired: 7 in, 1 out]
              }
              frame #1 {
                n122 = Unbundle By Name(w241) -> ("初始位置"=w240:refnum<vi>)
                n123 = property class="Bool"(reference=w240, "DisabledEnum"=T8."Enabled" ("禁用")) -> ()  [unwired: 1 in, 2 out]
              }
              frame #2 {
                w245 = 255
                n124 = call <vilib>:"RGB to Color.vi"("B"=u8 0 ("R"), "G"=w245, "R"=w245) -> ("Color"=w248:u32)
                n125 = Bundle("请点击初始位置", "Color"=w248) -> (w247:cluster{string, "Color":u32})  [unwired: 1 in]
                n126 = Enqueue Element(queue=w246, element=w247, error in (no error)=w243) -> (error out=w242:errorcluster)  [unwired: 1 in, 2 out]
                n127 = call <vilib>:"Clear Errors.vi"("error in (no error)"=w242) -> ()  [unwired: 5 in, 2 out]
              }
            }
            n128 = global read "参数.vi" "激光器状态"() -> (w233:T14)
            n129 = call <vilib>:"RGB to Color.vi"("B"=w225, "G"=u8 255 ("R"), "R"=w225) -> ("Color"=w229:u32)
            n130 = Bundle By Name(cluster=w233, "衰减片位置.近场相机位置"=衰减片电机位置枚举器."0倍") -> (w231:T14)
            n131 = Bundle("电机归0中", "Color"=w229) -> (w228:cluster{string, "Color":u32})  [unwired: 1 in]
            n132 = global write "参数.vi" "激光器状态"(w231) -> ()
            n133 = Enqueue Element(queue=w227, element=w228) -> (queue out=w224:refnum<queue>, error out=w222:errorcluster)  [unwired: 2 in, 1 out]
          }
          frame "CMD::InitPosition" {
            n134 = flat-sequence {
              tunnel: w256 -> [w265]
              tunnel: [w265] -> w255
              tunnel: [w264] -> w254
              tunnel: w253 -> [w264]
              tunnel: w252 -> [w258]
              tunnel: [w257] -> w251
              tunnel: w255 -> [w283]
              tunnel: w254 -> [w281]
              tunnel: w251 -> [w270]
              frame #0 {
                w259 = 0
                n135 = call <vilib>:"RGB to Color.vi"("B"=w259, "G"=u8 255 ("R"), "R"=w259) -> ("Color"=w262:u32)
                n136 = call "ControlMotor.vi"("控制电机指令"=控制电机指令枚举器."运动", "位置"=控制电机位置枚举器."近场相机") -> ()  [unwired: 6 in, 1 out]
                n137 = Bundle("电机运动中", "Color"=w262) -> (w261:cluster{string, "Color":u32})  [unwired: 1 in]
                n138 = Enqueue Element(queue=w258, element=w261) -> (queue out=w257:refnum<queue>)  [unwired: 2 in, 2 out]
              }
              frame #1 {
                w271 = 0
                w268 = T8."Enabled" ("禁用")
                n139 = Unbundle By Name(w283) -> ("衰减挡位"=w282:refnum<vi>)
                n140 = call <vilib>:"RGB to Color.vi"("B"=w271, "G"=u8 255 ("R"), "R"=w271) -> ("Color"=w274:u32)
                n141 = Unbundle By Name(w281) -> ("X"=w280:refnum<vi>, "Y"=w279:refnum<vi>, "Z"=w278:refnum<vi>, "旋转"=w277:refnum<vi>, "俯仰"=w276:refnum<vi>, "观察位置"=w269:refnum<vi>)
                n142 = property class="Clust"(reference=w280, "DisabledEnum"=w268) -> ()  [unwired: 1 in, 2 out]
                n143 = property class="Clust"(reference=w279, "DisabledEnum"=w268) -> ()  [unwired: 1 in, 2 out]
                n144 = property class="Clust"(reference=w278, "DisabledEnum"=w268) -> ()  [unwired: 1 in, 2 out]
                n145 = property class="Clust"(reference=w277, "DisabledEnum"=w268) -> ()  [unwired: 1 in, 2 out]
                n146 = property class="Clust"(reference=w276, "DisabledEnum"=w268) -> ()  [unwired: 1 in, 2 out]
                n147 = property class="Knob (严格)"(reference=w282, "DisabledEnum"=w268) -> ()  [unwired: 1 in, 2 out]
                n148 = Bundle("请开始调整", "Color"=w274) -> (w273:cluster{string, "Color":u32})  [unwired: 1 in]
                n149 = property class="Bool"(reference=w269, "DisabledEnum"=w268) -> ()  [unwired: 1 in, 2 out]
                n150 = Enqueue Element(queue=w270, element=w273) -> ()  [unwired: 2 in, 3 out]
              }
            }
          }
          frame "CMD::WritePostion" {
            n151 = call "ControlMotorDefinePostionParam.vi"() -> ("位置信息"=w287:T15)  [unwired: 11 in]
            n152 = call "ControlReadPulseAll.vi"() -> ("PosOut"=w285:dbl[])  [unwired: 3 in]
            n153 = Unbundle By Name(w287) -> ("近场相机"=w286:cluster{"控制电机":T13, "位置":dbl}[])
            n154 = for {
              tunnel: w286 -> [w294] mode=indexing
              tunnel: w285 -> [w293]
              tunnel: [w289] -> w284 mode=indexing
              n155 = Unbundle By Name(w294) -> ("控制电机"=w292:T13, "位置"=w291:dbl)
              n156 = Index Array(array=w293, index=w292) -> (element=w290:dbl)
              n157 = Subtract(x=w290, y=w291) -> (x-y=w289:dbl)
            }
            n158 = call "保存初始位置.vi"("PosDataIn"=w284) -> ()  [unwired: 11 in]
          }
          frame "MotorFoward" {
            n159 = Variant To Data(type=控制电机枚举器."Z" ("控制电机"), Variant=w299) -> (data=w295:T13)  [unwired: 1 in, 1 out]
            n160 = case shown="\"Z\", 默认" w295 {
              tunnel: [1.0 ("位置") 0.1 ("位置")] -> w297
              frame "Z", Default {
              }
              frame "俯仰", "旋转" {
              }
            }
            n161 = call "MotorMoveRelative.vi"("位置"=w297, "axis"=w295) -> ()  [unwired: 2 in, 1 out]
          }
          frame "MotorBackward" {
            n162 = Variant To Data(type=控制电机枚举器."Z" ("控制电机"), Variant=w303) -> (data=w305:T13)  [unwired: 1 in, 1 out]
            n163 = call "MotorMoveRelative.vi"("位置"=-1.0, "axis"=w305) -> ()  [unwired: 2 in, 1 out]
          }
          frame "MotorGoPostion" {
            n164 = Bundle("控制电机"=控制电机枚举器."Z", 0.0) -> (w312:cluster{"控制电机":T13, dbl})  [unwired: 1 in]
            n165 = Variant To Data(type=w312, Variant=w311) -> (data=w310:cluster{"控制电机":T13, dbl})  [unwired: 1 in, 1 out]
            n166 = Unbundle(w310) -> ("控制电机"=w309:T13, w308:dbl)
            n167 = call "MotorRotateInJoint.vi"("位置"=w308, "axis"=w309) -> ()  [unwired: 2 in, 1 out]
          }
        }
      }
      frame Error {
      }
    }
  }
  n168 = while "While循环" {
    shift-right: [w324] -> _
    shift-left: "Idle" -> [w326]
    tunnel: w30 -> [w323]
    shift-right: [w318] -> w10
    shift-left: T4 refnum ("IMAQdx Session Out") -> [w319]
    tunnel: w33 -> [w317]
    stop <- w325 stop-if-true
    # "相机采集"
    n169 = Get Queue Status(queue=w323) -> (queue out=w320:refnum<queue>, error out=w321:errorcluster, # elements in queue=w322:i32)  [unwired: 2 in, 5 out]
    n170 = case shown="无错误" w321 {
      tunnel: w326 -> [w330 w352]
      tunnel: [w336 TRUE] -> w325
      tunnel: [w335 w352] -> w324
      tunnel: w322 -> [w334 _]
      tunnel: w320 -> [w332 _]
      tunnel: w319 -> [w329 w353]
      tunnel: [w327 w353] -> w318
      tunnel: w317 -> [w328 _]
      frame No Error {
        n171 = Greater Than 0?(x=w334) -> (x > 0?=w333:bool)
        n172 = case shown="假" w333 {
          tunnel: w332 -> [_ w342]
          tunnel: [w338 w340] -> w331
          tunnel: [w337 w339] -> w327
          tunnel: w330 -> [w338 _]
          tunnel: w329 -> [w337 _]
          frame False {
          }
          frame True {
            n173 = Dequeue Element(queue=w342) -> (element=w341:cluster{"CMD":string, "IMAQdx Session Out":T4})  [unwired: 2 in, 3 out]
            n174 = Unbundle By Name(w341) -> ("CMD"=w340:string, "IMAQdx Session Out"=w339:T4)
          }
        }
        n175 = case shown="\"Capture\"" w331 {
          selector: w331 -> [w343 w350]
          tunnel: [_ FALSE] -> w336
          tunnel: [w343 w350] -> w335
          tunnel: w327 -> [_ w348]
          tunnel: w328 -> [_ w349]
          frame "Idle", Default {
          }
          frame "Capture" {
            n176 = call <vilib>:"IMAQdx Grab2.vi"("Image In"=w349, "Session In"=w348) -> ("error out"=w347:errorcluster, "Image Out"=w346:T2)  [unwired: 6 in, 2 out]
            n177 = call "Alligent_DrawOverLay.vi"("Image"=w346) -> ("Image Out"=w345:T2)  [unwired: 8 in, 2 out]
            "近场图" <- w345
            n178 = call <vilib>:"Clear Errors.vi"("error in (no error)"=w347) -> ()  [unwired: 5 in, 2 out]
            n179 = call "IMAQ Centroid"("Image"=w345) -> ("Centroid"=→"Centroid":cluster{"X Centroid":sgl, "Y Centroid":sgl})  [unwired: 3 in, 1 out]
          }
        }
      }
      frame Error {
      }
    }
  }
  n180 = control-ref of="Centroid"() -> (w2:refnum<vi>)
  n181 = while "While循环" {
    tunnel: w17 -> [w355]
    tunnel: [w355] -> w40
    tunnel: w13 -> [w359]
    tunnel: w30 -> [w358]
    tunnel: [w359] -> w29
    tunnel: [w358] -> w28
    tunnel: w3 -> [w357]
    tunnel: w2 -> [w356]
    stop <- w360 stop-if-true
    # "操作"
    n182 = event shown="[12] \"X.目标位置\": 值改变" {
      selector: _ -> [_ _ _ _ _ _ _ _ _ _ _ _ _ _ _ _ _ _ _ _ _ _ _ _ _]
      dyn-events: _ -> [_ _ _ _ _ _ _ _ _ _ _ _ _ _ _ _ _ _ _ _ _ _ _ _ _]
      timeout: 20 -> [_ _ _ _ _ _ _ _ _ _ _ _ _ _ _ _ _ _ _ _ _ _ _ _ _]
      tunnel: [_ _ TRUE w417 _ _ _ _ _ TRUE _ _ _ _ _ _ _ _ _ _ _ _ _ _ _] -> w360
      tunnel: w355 -> [_ w412 _ w416 w418 w420 w422 w428 w430 w437 w442 w443 w448 w453 w457 w462 w467 w471 w476 w481 w485 w490 w495 w499 w506]
      tunnel: w357 -> [w379 _ _ _ _ _ _ _ _ _ _ _ _ _ _ _ _ _ _ _ _ _ _ _ _]
      tunnel: w356 -> [w369 _ _ _ _ _ _ _ _ _ _ _ _ _ _ _ _ _ _ _ _ _ _ _ _]
      event Timeout {
        w374 = i16 2 ("精度(6)")
        (unwired) "" ("元素")
        w378 = i16 2 ("精度(6)")
        w397 = i16 2 ("精度(6)")
        n183 = event-data() -> ()  [unwired: 1 in, 3 out]
        n184 = call "ControlReadPulseAll.vi"() -> ("PosOut"=w392:dbl[])  [unwired: 3 in]
        n185 = global read "参数.vi" "激光器状态"() -> (w411:T14)
        n186 = Index Array(array=w392) -> (element #1=w391:dbl, element #2=w390:dbl, element #3=w389:dbl, element #4=w386:dbl, element #5=w388:dbl, element #6=w385:dbl)  [unwired: 6 in]
        n187 = Unbundle By Name(w411) -> ("衰减片位置.近场相机位置"=w382:T7)
        n188 = Number To Fractional String(number=w388, precision (6)=w397) -> (F-format string=w398:string)  [unwired: 2 in]
        n189 = Number To Fractional String(number=w385, precision (6)=w397) -> (F-format string=w399:string)  [unwired: 2 in]
        n190 = Number To Fractional String(number=w391, precision (6)=w378) -> (F-format string=w400:string)  [unwired: 2 in]
        n191 = Number To Fractional String(number=w390, precision (6)=w378) -> (F-format string=w401:string)  [unwired: 2 in]
        n192 = Number To Fractional String(number=w389, precision (6)=w378) -> (F-format string=w402:string)  [unwired: 2 in]
        n193 = Number To Fractional String(number=w386, precision (6)=w378) -> (F-format string=w387:string)  [unwired: 2 in]
        n194 = Number To Decimal String(number=w382) -> (decimal integer string=w381:string)  [unwired: 1 in]
        n195 = Build Array("衰减片位置", w381) -> (w380:string[])
        n196 = Build Array("位置 Z/mm", w400) -> (w404:string[])
        n197 = Build Array("位置 Y/mm", w401) -> (w405:string[])
        n198 = Build Array("位置 X/mm", w402) -> (w406:string[])
        n199 = Build Array("发散角位置 /mm", w387) -> (w393:string[])
        n200 = Build Array("俯仰 /°", w398) -> (w394:string[])
        n201 = Build Array("旋转 /°", w399) -> (w395:string[])
        n202 = property class="Clust (严格)"(reference=w369) -> ("Value"=w368:cluster{"X Centroid":sgl, "Y Centroid":sgl})  [unwired: 1 in, 2 out]
        n203 = Unbundle By Name(w368) -> ("X Centroid"=w366:sgl, "Y Centroid"=w364:sgl)
        n204 = Subtract(x=w364, y=sgl 291.0) -> (x-y=w362:sgl)
        n205 = Subtract(x=w366, y=sgl 391.0) -> (x-y=w367:sgl)
        n206 = Number To Fractional String(number=w362, precision (6)=w374) -> (F-format string=w372:string)  [unwired: 2 in]
        n207 = Build Array("中心点Y", w372) -> (w370:string[])
        n208 = Number To Fractional String(number=w367, precision (6)=w374) -> (F-format string=w373:string)  [unwired: 2 in]
        n209 = Build Array("中心点X", w373) -> (w371:string[])
        n210 = Build Array(w380, w406, w405, w404, w393, w395, w394, w371, w370) -> (w403:string[][])
        n211 = property on="属性节点" class="MCListbox (严格)"(reference=w379, "ItemNames"=w403, "ActiveCell"=T16 {"Row"=0, "Column"=0} ("活动单元格:活动单元格")) -> ()  [unwired: 1 in, 2 out]
      }
      event "观察位置": Value Change {
        n212 = event-data() -> ()  [unwired: 1 in, 6 out]
        n213 = Enqueue Element(queue=w412, element=cluster{"Data":variant, "CMD":string} {"Data"=variant, "CMD"="CMD::EstimatePositon"} ("元素")) -> ()  [unwired: 2 in, 3 out]
      }
      event Panel Close {
        n214 = event-data() -> ()  [unwired: 1 in, 4 out]
      }
      event "退出": Value Change {
        n215 = event-data() -> ("NewVal"=w417:bool)  [unwired: 1 in, 5 out]
        n216 = Enqueue Element(queue=w416, element=cluster{"Data":variant, "CMD":string} {"Data"=variant, "CMD"="CMD::exit"} ("元素")) -> ()  [unwired: 2 in, 3 out]
      }
      event "链接相机": Value Change {
        n217 = event-data() -> ()  [unwired: 1 in, 6 out]
        n218 = Enqueue Element(queue=w418, element=cluster{"Data":variant, "CMD":string} {"Data"=variant, "CMD"="CMD::ConnectCam"} ("元素")) -> ()  [unwired: 2 in, 3 out]
      }
      event "链接电机": Value Change {
        n219 = event-data() -> ()  [unwired: 1 in, 6 out]
        n220 = Enqueue Element(queue=w420, element=cluster{"Data":variant, "CMD":string} {"Data"=variant, "CMD"="CMD::ConnectMotor"} ("元素")) -> ()  [unwired: 2 in, 3 out]
      }
      event "初始位置": Value Change {
        n221 = event-data() -> ()  [unwired: 1 in, 6 out]
        n222 = Enqueue Element(queue=w422, element=cluster{"Data":variant, "CMD":string} {"Data"=variant, "CMD"="CMD::InitPosition"} ("元素")) -> ()  [unwired: 2 in, 3 out]
      }
      event Value Change {
        n223 = event-data() -> ("NewVal"=w427:T1)  [unwired: 1 in, 5 out]
        n224 = To Variant(anything=w427) -> (Variant=w425:variant)
        n225 = Bundle("Variant"=w425, "CMD"="CMD::AttentorChange") -> (w424:cluster{"Variant":variant, "CMD":string})  [unwired: 1 in]
        n226 = Enqueue Element(queue=w428, element=w424) -> ()  [unwired: 2 in, 3 out]
      }
      event "相机曝光时间/ms": Value Change {
        n227 = event-data() -> ("NewVal"=w429:dbl)  [unwired: 1 in, 5 out]
        n228 = To Variant(anything=w429) -> (Variant=w432:variant)
        n229 = Bundle("Variant"=w432, "CMD"="CMD::ExposureTimeChange") -> (w431:cluster{"Variant":variant, "CMD":string})  [unwired: 1 in]
        n230 = Enqueue Element(queue=w430, element=w431) -> ()  [unwired: 2 in, 3 out]
      }
      event "记录位置": Value Change {
        n231 = event-data() -> ()  [unwired: 1 in, 6 out]
        n232 = Enqueue Element(queue=w437, element=cluster{"Data":variant, "CMD":string} {"Data"=variant, "CMD"="CMD::WritePostion"} ("元素")) -> (queue out=w436:refnum<queue>)  [unwired: 2 in, 2 out]
        n233 = Enqueue Element(queue=w436, element=cluster{"Data":variant, "CMD":string} {"Data"=variant, "CMD"="CMD::exit"} ("元素")) -> ()  [unwired: 2 in, 3 out]
      }
      event "X.前进1mm": Value Change {
        n234 = event-data() -> ()  [unwired: 1 in, 6 out]
        n235 = Bundle("控制电机"=控制电机枚举器."X", "CMD"="MotorFoward") -> (w439:cluster{"控制电机":T13, "CMD":string})  [unwired: 1 in]
        n236 = Enqueue Element(queue=w442, element=w439) -> ()  [unwired: 2 in, 3 out]
      }
      event "X.后退1mm": Value Change {
        n237 = event-data() -> ()  [unwired: 1 in, 6 out]
        n238 = Bundle("控制电机"=控制电机枚举器."X", "CMD"="MotorBackward") -> (w444:cluster{"控制电机":T13, "CMD":string})  [unwired: 1 in]
        n239 = Enqueue Element(queue=w443, element=w444) -> ()  [unwired: 2 in, 3 out]
      }
      event "X.目标位置": Value Change {
        n240 = event-data() -> ("NewVal"=w447:dbl)  [unwired: 1 in, 5 out]
        n241 = Bundle("控制电机"=控制电机枚举器."X", "NewVal"=w447) -> (w449:cluster{"控制电机":T13, "NewVal":dbl})  [unwired: 1 in]
        n242 = Bundle(w449, "CMD"="MotorGoPostion") -> (w451:T17)  [unwired: 1 in]
        n243 = Enqueue Element(queue=w448, element=w451) -> ()  [unwired: 2 in, 3 out]
      }
      event "Y.前进1mm": Value Change {
        n244 = event-data() -> ()  [unwired: 1 in, 6 out]
        n245 = Bundle("控制电机"=控制电机枚举器."Y", "CMD"="MotorFoward") -> (w454:cluster{"控制电机":T13, "CMD":string})  [unwired: 1 in]
        n246 = Enqueue Element(queue=w453, element=w454) -> ()  [unwired: 2 in, 3 out]
      }
      event "Y.后退1mm": Value Change {
        n247 = event-data() -> ()  [unwired: 1 in, 6 out]
        n248 = Bundle("控制电机"=控制电机枚举器."Y", "CMD"="MotorBackward") -> (w458:cluster{"控制电机":T13, "CMD":string})  [unwired: 1 in]
        n249 = Enqueue Element(queue=w457, element=w458) -> ()  [unwired: 2 in, 3 out]
      }
      event "Y.目标位置": Value Change {
        n250 = event-data() -> ("NewVal"=w461:dbl)  [unwired: 1 in, 5 out]
        n251 = Bundle("控制电机"=控制电机枚举器."Y", "NewVal"=w461) -> (w463:cluster{"控制电机":T13, "NewVal":dbl})  [unwired: 1 in]
        n252 = Bundle(w463, "CMD"="MotorGoPostion") -> (w465:T17)  [unwired: 1 in]
        n253 = Enqueue Element(queue=w462, element=w465) -> ()  [unwired: 2 in, 3 out]
      }
      event "Z.前进1mm": Value Change {
        n254 = event-data() -> ()  [unwired: 1 in, 6 out]
        n255 = Bundle("控制电机"=控制电机枚举器."Z", "CMD"="MotorFoward") -> (w468:cluster{"控制电机":T13, "CMD":string})  [unwired: 1 in]
        n256 = Enqueue Element(queue=w467, element=w468) -> ()  [unwired: 2 in, 3 out]
      }
      event "Z.后退1mm": Value Change {
        n257 = event-data() -> ()  [unwired: 1 in, 6 out]
        n258 = Bundle("控制电机"=控制电机枚举器."Z", "CMD"="MotorBackward") -> (w472:cluster{"控制电机":T13, "CMD":string})  [unwired: 1 in]
        n259 = Enqueue Element(queue=w471, element=w472) -> ()  [unwired: 2 in, 3 out]
      }
      event "Z.目标位置": Value Change {
        n260 = event-data() -> ("NewVal"=w475:dbl)  [unwired: 1 in, 5 out]
        n261 = Bundle("控制电机"=控制电机枚举器."Z", "NewVal"=w475) -> (w477:cluster{"控制电机":T13, "NewVal":dbl})  [unwired: 1 in]
        n262 = Bundle(w477, "CMD"="MotorGoPostion") -> (w479:T17)  [unwired: 1 in]
        n263 = Enqueue Element(queue=w476, element=w479) -> ()  [unwired: 2 in, 3 out]
      }
      event Value Change {
        n264 = event-data() -> ()  [unwired: 1 in, 6 out]
        n265 = Bundle("控制电机"=控制电机枚举器."旋转", "CMD"="MotorFoward") -> (w482:cluster{"控制电机":T13, "CMD":string})  [unwired: 1 in]
        n266 = Enqueue Element(queue=w481, element=w482) -> ()  [unwired: 2 in, 3 out]
      }
      event Value Change {
        n267 = event-data() -> ()  [unwired: 1 in, 6 out]
        n268 = Bundle("控制电机"=控制电机枚举器."旋转", "CMD"="MotorBackward") -> (w486:cluster{"控制电机":T13, "CMD":string})  [unwired: 1 in]
        n269 = Enqueue Element(queue=w485, element=w486) -> ()  [unwired: 2 in, 3 out]
      }
      event Value Change {
        n270 = event-data() -> ("NewVal"=w489:dbl)  [unwired: 1 in, 5 out]
        n271 = Bundle("控制电机"=控制电机枚举器."旋转", "NewVal"=w489) -> (w491:cluster{"控制电机":T13, "NewVal":dbl})  [unwired: 1 in]
        n272 = Bundle(w491, "CMD"="MotorGoPostion") -> (w493:T17)  [unwired: 1 in]
        n273 = Enqueue Element(queue=w490, element=w493) -> ()  [unwired: 2 in, 3 out]
      }
      event "俯仰.前进0.1": Value Change {
        n274 = event-data() -> ()  [unwired: 1 in, 6 out]
        n275 = Bundle("控制电机"=控制电机枚举器."俯仰", "CMD"="MotorFoward") -> (w496:cluster{"控制电机":T13, "CMD":string})  [unwired: 1 in]
        n276 = Enqueue Element(queue=w495, element=w496) -> ()  [unwired: 2 in, 3 out]
      }
      event "俯仰.后退0.1": Value Change {
        n277 = event-data() -> ()  [unwired: 1 in, 6 out]
        n278 = Bundle("控制电机"=控制电机枚举器."俯仰", "CMD"="MotorBackward") -> (w500:cluster{"控制电机":T13, "CMD":string})  [unwired: 1 in]
        n279 = Enqueue Element(queue=w499, element=w500) -> ()  [unwired: 2 in, 3 out]
      }
      event "俯仰.目标位置": Value Change {
        n280 = event-data() -> ("NewVal"=w504:dbl)  [unwired: 1 in, 5 out]
        n281 = Bundle("控制电机"=控制电机枚举器."俯仰", "NewVal"=w504) -> (w503:cluster{"控制电机":T13, "NewVal":dbl})  [unwired: 1 in]
        n282 = Bundle(w503, "CMD"="MotorGoPostion") -> (w507:T17)  [unwired: 1 in]
        n283 = Enqueue Element(queue=w506, element=w507) -> ()  [unwired: 2 in, 3 out]
      }
    }
  }
  n284 = Release Queue(queue=w28) -> ()  [unwired: 2 in, 3 out]
  n285 = Release Queue(queue=w29) -> ()  [unwired: 2 in, 3 out]
  n286 = Release Queue(queue=w40) -> ()  [unwired: 2 in, 3 out]
  n287 = call <vilib>:"IMAQdx Close Camera.vi"("Session In"=w10) -> ("error out"=w9:errorcluster)  [unwired: 10 in]
  n288 = call <vilib>:"Clear Errors.vi"("error in (no error)"=w9) -> ()  [unwired: 5 in, 2 out]
